vi "Read NI 9228.vi"(8 "error in":errorcluster, 11 "NI 9228 in":refnum<class "NI 9228.lvclass">) -> (0 "error out":errorcluster, 1 "channel settings":T1[](array[typedef]), 2 "conversion time":T2, 3 "NI 9228 out":refnum<class "NI 9228.lvclass">)   [LabVIEW 2017, in "Scan Engine Scripting.lvlib" / "NI 9228.lvclass"]
uses:
  NI 9228.lvclass
  Mode Classes/Analog Inputs with Conversion Time Mode/Conversion Time.ctl
  Mode Classes/Controls/analog channel settings.ctl
  Mode Classes/Analog Inputs with Conversion Time Mode/Analog Input with Conversion Time Mode.lvclass
  Scan Engine Scripting.lvlib
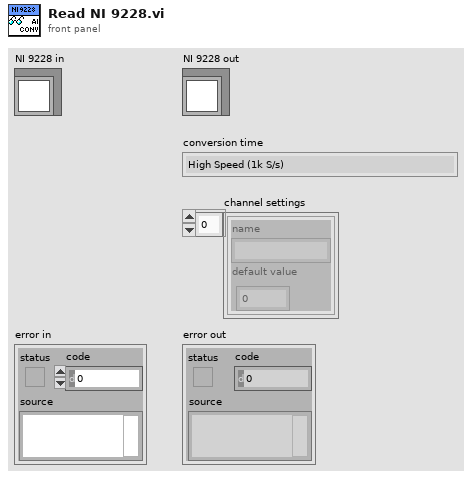
[diagram p1: front panel]
types:
  T1 = typedef "Scan Engine Scripting.lvlib/analog channel settings.ctl" = cluster{"name":string, "default value":dbl}
  T2 = typedef "Scan Engine Scripting.lvlib/Analog Input with Conversion Time Mode.lvclass/Conversion Time.ctl" = enum16{"High Speed (1k S/s)", "Medium Speed (100 S/s)", "Medium Resolution (50/60Hz Rejection - 12 S/s)", "High Resolution (50/60Hz Rejection - 2 S/s)"}
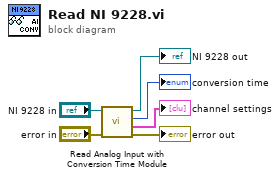
[diagram p0: block diagram]
diagram:
  n1 = call-dynamic "Read Analog Input with Conversion Time Module.vi"("error in"="error in", "module in"="NI 9228 in") -> ("error out"=→"error out":errorcluster, "channel settings"=→"channel settings":T1[], "conversion time"=→"conversion time":T2, "module out"=→"NI 9228 out":refnum<class "NI 9228.lvclass">)  [unwired: 6 in]
